vi "GetForceTrigger.vi"(8 "error in":errorcluster, 10 "status":variant, 11 "data group":string) -> (0 "error out":errorcluster, 3 "force trigger":bool)   [LabVIEW 2017, in "Trigger.lvlib"]
uses:
  <vilib>/addons/InsightCM/Devices/Shared/Common/Trigger/Trigger.lvlib
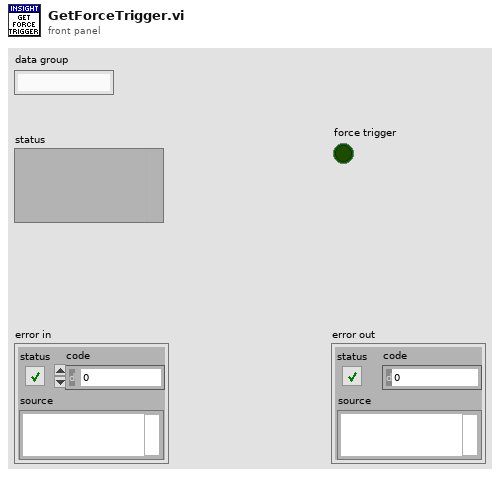
[diagram p1: front panel]
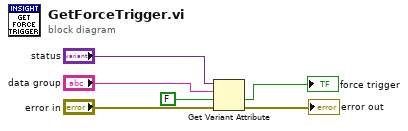
[diagram p0: block diagram]
diagram:
  n1 = Get Variant Attribute(Variant="status", name="data group", default value (empty Variant)=FALSE ("force trigger"), error in="error in") -> (value=→"force trigger":bool, error out=→"error out":errorcluster)  [unwired: 2 out]
